vi "QVA_GetAttributeNames.vi"(0 "QueueIn":refnum<queue>, 3 "Timeout [ms]":i32=-1, 5 "ErrorIn":errorcluster) -> (14 "QueueOut":refnum<queue>, 16 "ok":bool, 17 "DataArray":T1(array[cluster]), 18 "Names":string[](array[string]), 19 "ErrorOut":errorcluster)   [LabVIEW 2016]
doc: "Gibt alle Namen und Values eines Single Element Queue Variant Attributes aus.\n\nsige / 3.12.13"
uses:
  private/QVA.VariableDataTypeDef.ctl
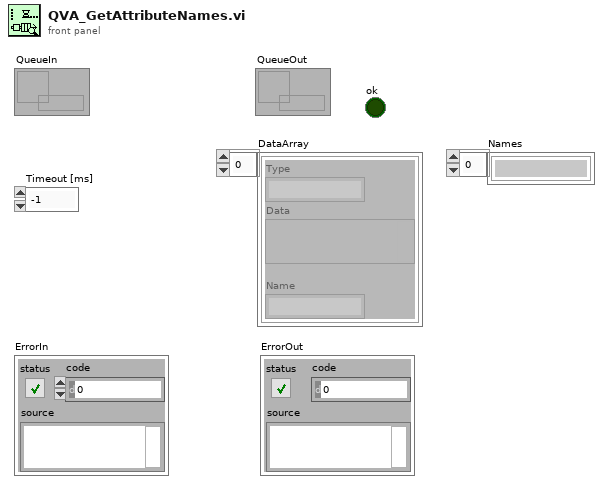
[diagram p1: front panel]
types:
  T1 = cluster{"Type":string, "Data":variant, "Name":string}[]
  T2 = typedef "QVA.VariableDataTypeDef.ctl" = cluster{"Type":string, "Data":variant}
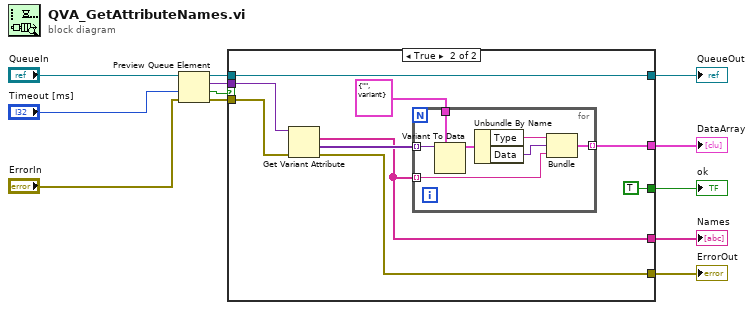
[diagram p0: block diagram]
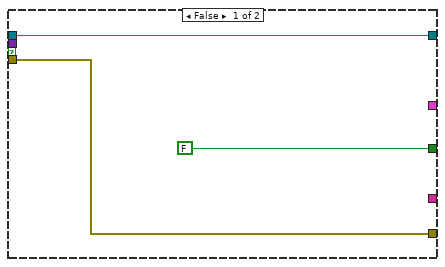
[diagram p2: hidden frame]
diagram:
  n1 = Preview Queue Element(queue="QueueIn", timeout in ms (-1)="Timeout [ms]", error in (no error)="ErrorIn") -> (queue out=w4:refnum<queue>, element=w8:variant, timed out?=w5:bool, error out=w9:errorcluster)
  n2 = case shown="True" w5 {
    tunnel: w9 -> [w14 w24]
    tunnel: w8 -> [_ w23]
    tunnel: [w14 w22] -> w7
    tunnel: [FALSE TRUE] -> w6
    tunnel: w4 -> [w15 w21]
    tunnel: [w15 w21] -> w3
    tunnel: [_ w18] -> w2
    tunnel: [_ w17] -> w1
    frame False {
    }
    frame True {
      n3 = Get Variant Attribute(Variant=w23, error in=w24) -> (names=w17:string[], values=w20:variant[], error out=w22:errorcluster)  [unwired: 2 in, 1 out]
      n4 = for {
        tunnel: w20 -> [w31] mode=indexing
        tunnel: T2 {"Type"="", "Data"=variant} -> [w29]
        tunnel: w17 -> [w25] mode=indexing
        tunnel: [w26] -> w18 mode=indexing
        n5 = Variant To Data(type=w29, Variant=w31) -> (data=w30:T2)  [unwired: 1 in, 1 out]
        n6 = Unbundle By Name(w30) -> ("Type"=w28:string, "Data"=w27:variant)
        n7 = Bundle("Type"=w28, "Data"=w27, w25) -> (w26:cluster{"Type":string, "Data":variant, string})  [unwired: 1 in]
      }
    }
  }
  "QueueOut" <- w3
  "ErrorOut" <- w7
  "ok" <- w6
  "DataArray" <- w2
  "Names" <- w1
